vi "Get - Matrix - Reals.vi"(5 "use temporary file?":bool, 7 "data type of variable":dbl[][](array[numeric]), 8 "error in":errorcluster, 10 "variable name":string, 11 "pipe in":T1) -> (0 "error out":errorcluster, 2 "value":dbl[][](array[numeric]) format="%.2f", 3 "pipe out":T1)   [LabVIEW 2013, in "GOLPI library.lvlib"]
uses:
  GOLPI library.lvlib
  LV Process.lvlibp/Pipe Handle.ctl
  Custom Error Codes Enum Type Def.vi
  LV Process.lvlibp
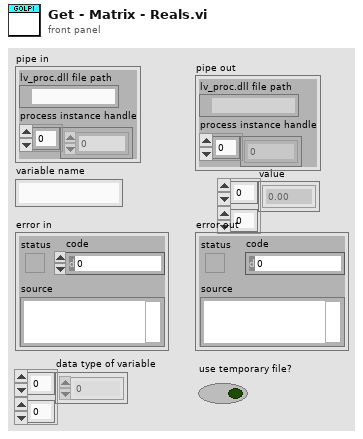
[diagram p1: front panel]
types:
  T1 = typedef "LV Process.lvlibp/Pipe Handle.ctl" = cluster{"lv_proc.dll file path":path, "process instance handle":u32[]}
  T2 = typedef "GOLPI library.lvlib/Custom Error Codes Enum Type Def.vi" = enum16{"no error", "00 working directory PAR1 missing", "01 octave binary PAR1 missing", "02 octave report error PAR1", "03 empty output last cmd PAR1", "04 missing temporary file PAR1", "10 var PAR1 not string", "11 var PAR1 not num, scal, ~compl", "12 var PAR1 not num, scal, compl", "13 var PAR1 not num, vect, ~compl", "14 var PAR1 not num, vect, compl", "15 var PAR1 not num, mat, ~compl", "16 var PAR1 not num, mat, ~compl", "99 not finished"}
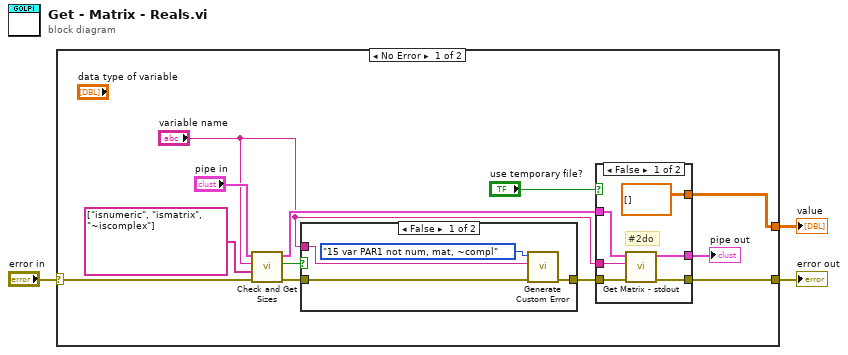
[diagram p0: block diagram]
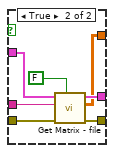
[diagram p2: hidden frame]
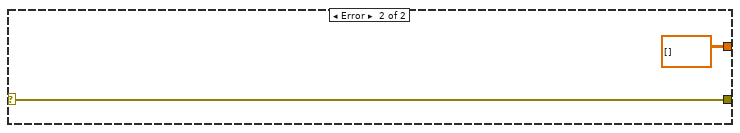
[diagram p4: hidden frame]
diagram:
  n1 = case shown="No Error" "error in" {
    selector: "error in" -> [w12 w35]
    tunnel: [w6 w35] -> w3
    tunnel: [w15 dbl[][] [] ("double array")] -> w1
    frame No Error {
      n2 = call "Check and Get Sizes.vi"("error in (no error)"=w12, "test commands"=string[] ["isnumeric", "ismatrix", "~iscomplex"], "variable name"="variable name", "pipe in"="pipe in") -> ("error out"=w11:errorcluster, "all tests OK?"=w13:bool, "pipe out"=w9:T1)  [unwired: 4 in, 1 out]
      n3 = case shown="False" w13 {
        tunnel: w11 -> [w31 w33]
        tunnel: [w30 w33] -> w7
        tunnel: "variable name" -> [w29 _]
        frame False {
          n4 = call "Generate Custom Error.vi"("error in"=w31, "PAR1"=w29, "Enum"=Custom_Error_Codes_Enum_Type_Def.vi."15 var PAR1 not num, mat, ~compl") -> ("error out"=w30:errorcluster)  [unwired: 8 in]
        }
        frame True {
        }
      }
      n5 = case shown="False" "use temporary file?" {
        tunnel: [dbl[][] [] ("double array") w22] -> w15
        tunnel: w9 -> [w18 w27]
        tunnel: [w17 w26] -> w8
        tunnel: w7 -> [w20 w24]
        tunnel: [w19 w23] -> w6
        tunnel: "variable name" -> [w16 w25]
        frame False {
          # "#2do"
          n6 = call "Get Matrix - stdout.vi"("error in (no error)"=w20, "variable name"=w16, "pipe in"=w18) -> ("error out"=w19:errorcluster, "pipe out"=w17:T1)  [unwired: 6 in, 1 out]
        }
        frame True {
          n7 = call "Get Matrix - file.vi"("is string"=FALSE, "error in (no error)"=w24, "variable name"=w25, "pipe in"=w27) -> ("error out"=w23:errorcluster, "double array"=w22:dbl[][], "pipe out"=w26:T1)  [unwired: 3 in, 2 out]
        }
      }
      "pipe out" <- w8
    }
    frame Error {
    }
  }
  "value" <- w1
  "error out" <- w3
